vi "DAQ.vi"() -> ()   [LabVIEW 2018]
uses:
  <vilib>/Platform/TimedLoop/XDataNode/timing_clust.ctl
  <vilib>/Platform/TimedLoop/XDataNode/nitl_modes.ctl
  <vilib>/Platform/TimedLoop/XDataNode/wakeup.ctl
  <vilib>/Analysis/baseanly.llb/Mean (DBL).vi
  <vilib>/FPGAPlugInAG/myRIO-1900/niLvFpga_Open_myRIO-1900.vi
  <vilib>/rvi/interface/common/dynamic/niFpgaDynamicAddResources.vi
  <vilib>/Utility/error.llb/Error Cluster From Error Code.vi
  <vilib>/rvi/errors/niLvFpgaAdjustHostInterfaceError.vi
  <vilib>/FPGAPlugInAG/Dynamic/niLvFpga_Close_Dynamic.vi
  <vilib>/rvi/interface/nirviOpenFPGA/nirviOpenFPGA.xnode
  FPGA Bitfiles/FirstTrial_FPGATarget_FPGAMain_Binary_Stochastic_DIO.lvbitx
  <vilib>/rvi/interface/nirviReadWriteControl/nirviReadWriteControl.xnode
  <vilib>/rvi/interface/nirviMethod/nirviMethod.xnode
  <vilib>/Platform/TimedLoop/XDataNode/XDataNode.xnode
  <vilib>/rvi/interface/nirviCloseFPGA/nirviCloseFPGA.xnode
  <vilib>/rvi/errors/niLvFpgaMergeErrorWithErrorCode.vi
  <vilib>/rvi/interface/Simulation/niFpgaSimulationCallBeginRW.vi
  <vilib>/Platform/TimedLoop/XDataNode/XDNodeRunTimeDep.lvlib
  <vilib>/Analysis/NI_AALBase.lvlib
  <vilib>/FPGAPlugInAG/Dynamic/niLvFpga_ReadFifo_Dynamic.vi
  NiFpgaLv.dll
  <vilib>/FPGAPlugInAG/Dynamic/niLvFpga_StartFifo_Dynamic.vi
  <vilib>/FPGAPlugInAG/Dynamic/niLvFpga_StopFifo_Dynamic.vi
panel:
  in  "Acquisitions":T1(tab)=enum."Recorded"
  out "Real Time Actuation Mean Chart":dbl(graph)=2.577495574951172
  out "Real Time Measurement Mean Chart":dbl(graph)=2.4726343154907227
  out "Measurement Data":i16[](array[numeric])=[754, 1268, 1779, 2292, 2798, 3300, 3794, 4083, 4089, 4094, 4094, 4095, 4093, 4095, 4094, 4095, 4094, 4095, 4093, 4095, 4093, 4094, 4093, 4095, 4093, 4095, 4093, 4095, 4093, 4095, 4093, 4095, 4093, 4095, 4093, 4095, 4092, 4095, 4092, 4095, 4092, 4095, 4092, 4095, 4093, 4095, 4094, 4095, 4094, 4095, 4094, 4095, 4094, 4095, 4095, 4095, 4094, 4095, 4094, 4094, 3947, 3428, 2884, 2343, 1812, 1284, 760, 250, 10, 8, 5, 5, 4, 4, 5, 5, 5, 5, 5, 4, 5, 5, 5, 4, 5, 4, 5, 5, 5, 5, 5, 5, 5, 4, 5, 5, 5, 5, 4, 5, 4, 5, 5, 5, 5, 4, 4, 5, 5, 5, 5, 5, 4, 5, 5, 5, 4, 5, 5, 5, 5, 5, 5, 136, 636, 1150, 1662, 2175, 2682, 3186, 3680, 4088, 4089, 4093, 4093, 4095, 4094, 4095, 4093, 4095, 4094, 4095, 4093, 4094, 4093, 4095, 4093, 4094, 4093, 4095, 4093, 4095, 4094, 4095, 4094, 4095, 4093, 4095, 4093, 4095, 4093, 4095, 4092, 4095, 4092, 4095, 4092, 4095, 4093, 4095, 4094, 4095, 4093, 4095, 4094, 4095, 4094, 4095, 4094, 4095, 4094, 4095, 4094, 4095, 4060, 3570, 3029, 2485, 1952, 1423, 897, 382, 4, 9, 6, 5, 4, 4, 5, 5, 5, 5, 4, 4, 4, 5, 5, 4, 5, 5, 5, 5, 5, 5, 5, 5, 4, 5, 5, 5, 5, 5, 5, 4, 5, 5, 5, 4, 4, 4, 5, 5, 5, 5, 5, 5, 5, 5, 5, 5, 5, 4, 5, 5, 5, 5, 5, 7, 500, 1013, 1526, 2037, 2548, 3052, 3550, 4034]
  out "Actuation Data":i16[](array[numeric])=[4095, 4095, 4095, 4095, 4095, 4095, 4095, 4095, 4095, 4095, 4095, 4095, 4095, 4095, 4095, 4095, 4095, 4095, 4095, 4095, 4095, 4095, 4095, 4095, 4095, 4095, 4095, 4095, 4095, 4095, 4095, 4095, 4095, 4095, 4095, 4095, 4095, 4095, 4095, 4095, 4095, 4095, 4095, 4095, 4095, 4095, 4095, 4095, 4095, 4095, 4095, 4095, 4095, 4095, 4095, 4095, 4095, 4095, 4095, 0, 0, 0, 0, 0, 0, 0, 0, 0, 0, 0, 0, 0, 0, 0, 0, 0, 0, 0, 0, 0, 0, 0, 0, 0, 0, 0, 0, 0, 0, 0, 0, 0, 0, 0, 0, 0, 0, 0, 0, 0, 0, 0, 0, 0, 0, 0, 0, 0, 0, 0, 0, 0, 0, 0, 0, 0, 0, 0, 0, 0, 0, 4095, 4095, 4095, 4095, 4095, 4095, 4095, 4095, 4095, 4095, 4095, 4095, 4095, 4095, 4095, 4095, 4095, 4095, 4095, 4095, 4095, 4095, 4095, 4095, 4095, 4095, 4095, 4095, 4095, 4095, 4095, 4095, 4095, 4095, 4095, 4095, 4095, 4095, 4095, 4095, 4095, 4095, 4095, 4095, 4095, 4095, 4095, 4095, 4095, 4095, 4095, 4095, 4095, 4095, 4095, 4095, 4095, 4095, 4095, 4095, 4095, 4095, 0, 0, 0, 0, 0, 0, 0, 0, 0, 0, 0, 0, 0, 0, 0, 0, 0, 0, 0, 0, 0, 0, 0, 0, 0, 0, 0, 0, 0, 0, 0, 0, 0, 0, 0, 0, 0, 0, 0, 0, 0, 0, 0, 0, 0, 0, 0, 0, 0, 0, 0, 0, 0, 0, 0, 0, 0, 0, 0, 0, 0, 0, 4095, 4095, 4095, 4095, 4095, 4095, 4095, 4095, 4095, 4095, 4095]
  out "Mean Measurement":dbl=2.4726343154907227 format="%0.2f"
  out "Mean Acatuation":dbl=2.577495574951172 format="%0.2f"
  out "Elements Remaining":u32=192
  out "Actuation Graph":waveform(i16)(graph)={"t0"=timestamp(0 s since 1904-01-01), "dt"=2.0, "Y"=array[3392 elements]}
  out "Measurement Graph":waveform(i16)(graph)={"t0"=timestamp(0 s since 1904-01-01), "dt"=2.0, "Y"=array[3520 elements]}
  out "Data File Path":path=path "c:/ni-rt/startup/03_11_16_04:11 PMTrial.csv"
  out "Sample Each Cycle":i32[](array[numeric])=[0, 0, 512, 960, 576, 384, 256, 192, 256, 256]
  out "Total Data Points":i32=3392
  in  "Settings":enum32{"Controls", "Logging Setting"}(tab)
  in  "Actuation Period (muS)":u32=5
  in  "Acquisition Period (muS)":u32=2
  in  "RT Period(muS)":i64=500
  in  "Recording Time (muS)":i64=5000
  in  "Signal Control":T2={"Mode"=enum."Square Wave", "Frequency (Periods/tick)"=0.0001005989033728838, "Phase (period)"=0.0} {"Frequency (Periods/tick)" format="%#_6f"}
  out "Frequency (kHz)":dbl=4.023956134915352
  in  "High Pass?":bool
  in  "Low Pass?":bool
  in  "Data File Name Label":string="Trial"
  in  "Continuous?":bool
  in  "Log Data?":bool
  out "Logging Progress":dbl(slide) scale=0.0..100.0
  out "Logging?":bool
  out "Finished Late? [i-1]":bool
  out "FIFO Timed Out?":bool
  in  "stop":bool
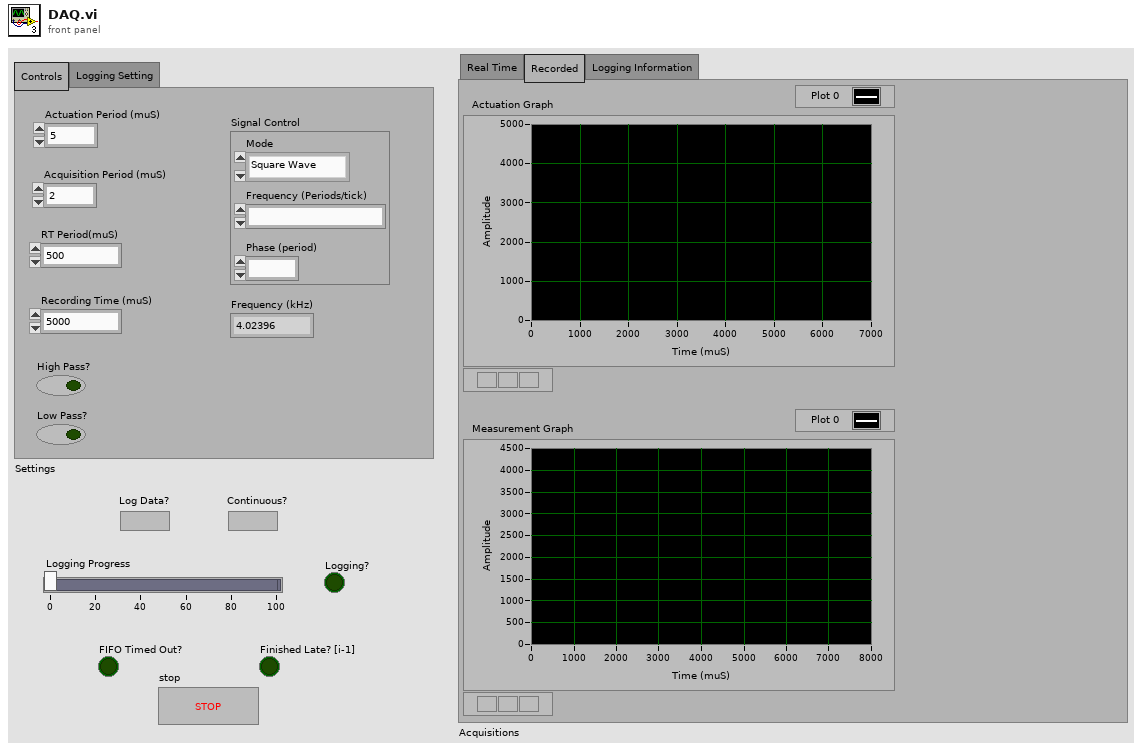
[diagram p1: front panel]
types:
  T1 = enum32{"Real Time", "Recorded", "Logging Information"}
  T2 = cluster{"Mode":enum16{"Square Wave", "Sine Wave", "White Noise", "Stochastic"}, "Frequency (Periods/tick)":fxp<+,32,0>, "Phase (period)":fxp<+,32,0>}
  T3 = typedef "XDNodeRunTimeDep.lvlib/timing_clust.ctl" = cluster{"Expected End [f-1]":u64, "Actual End [f-1]":u64, "Finished Late? [f-1]":bool, "Expected End [i-1]":u64, "Actual End [i-1]":u64, "Finished Late? [i-1]":bool, "Expected Start [i]":u64, "Actual Start [i]":u64, "Expected Start [f]":u64, "Actual Start [f]":u64, "Source Name":string, "Structure Name":string, "Period":i64, "Deadline":i64, "Offset":i64, "Start":i64, "Priority":i32, "Timeout":i32, "Mode":T4, "Wakeup Reason":T5, "Error":errorcluster, "Source Type":string, "Secondary Source Type":string, "Global End Time":u64, "Global Start Time":u64, "Frame Duration":u64, "Iteration Duration":u64, "Assigned CPU":i32, "I/O Scan Engine Mode":u32}
  T4 = typedef "XDNodeRunTimeDep.lvlib/nitl_modes.ctl" = enum32{"No Change", "Process missed periods, maintain original phase", "Discard missed periods, maintain original phase", "Process missed periods, ignore original phase", "Discard missed periods, ignore original phase"}
  T5 = typedef "XDNodeRunTimeDep.lvlib/wakeup.ctl" = enum32{"Normal", "Aborted", "Asynchronous wakeup", "Timing source error", "Timed loop error", "Timeout"}
  T6 = enum16{"open", "replace", "create", "open or create", "replace or create", "replace or create with confirmation"}
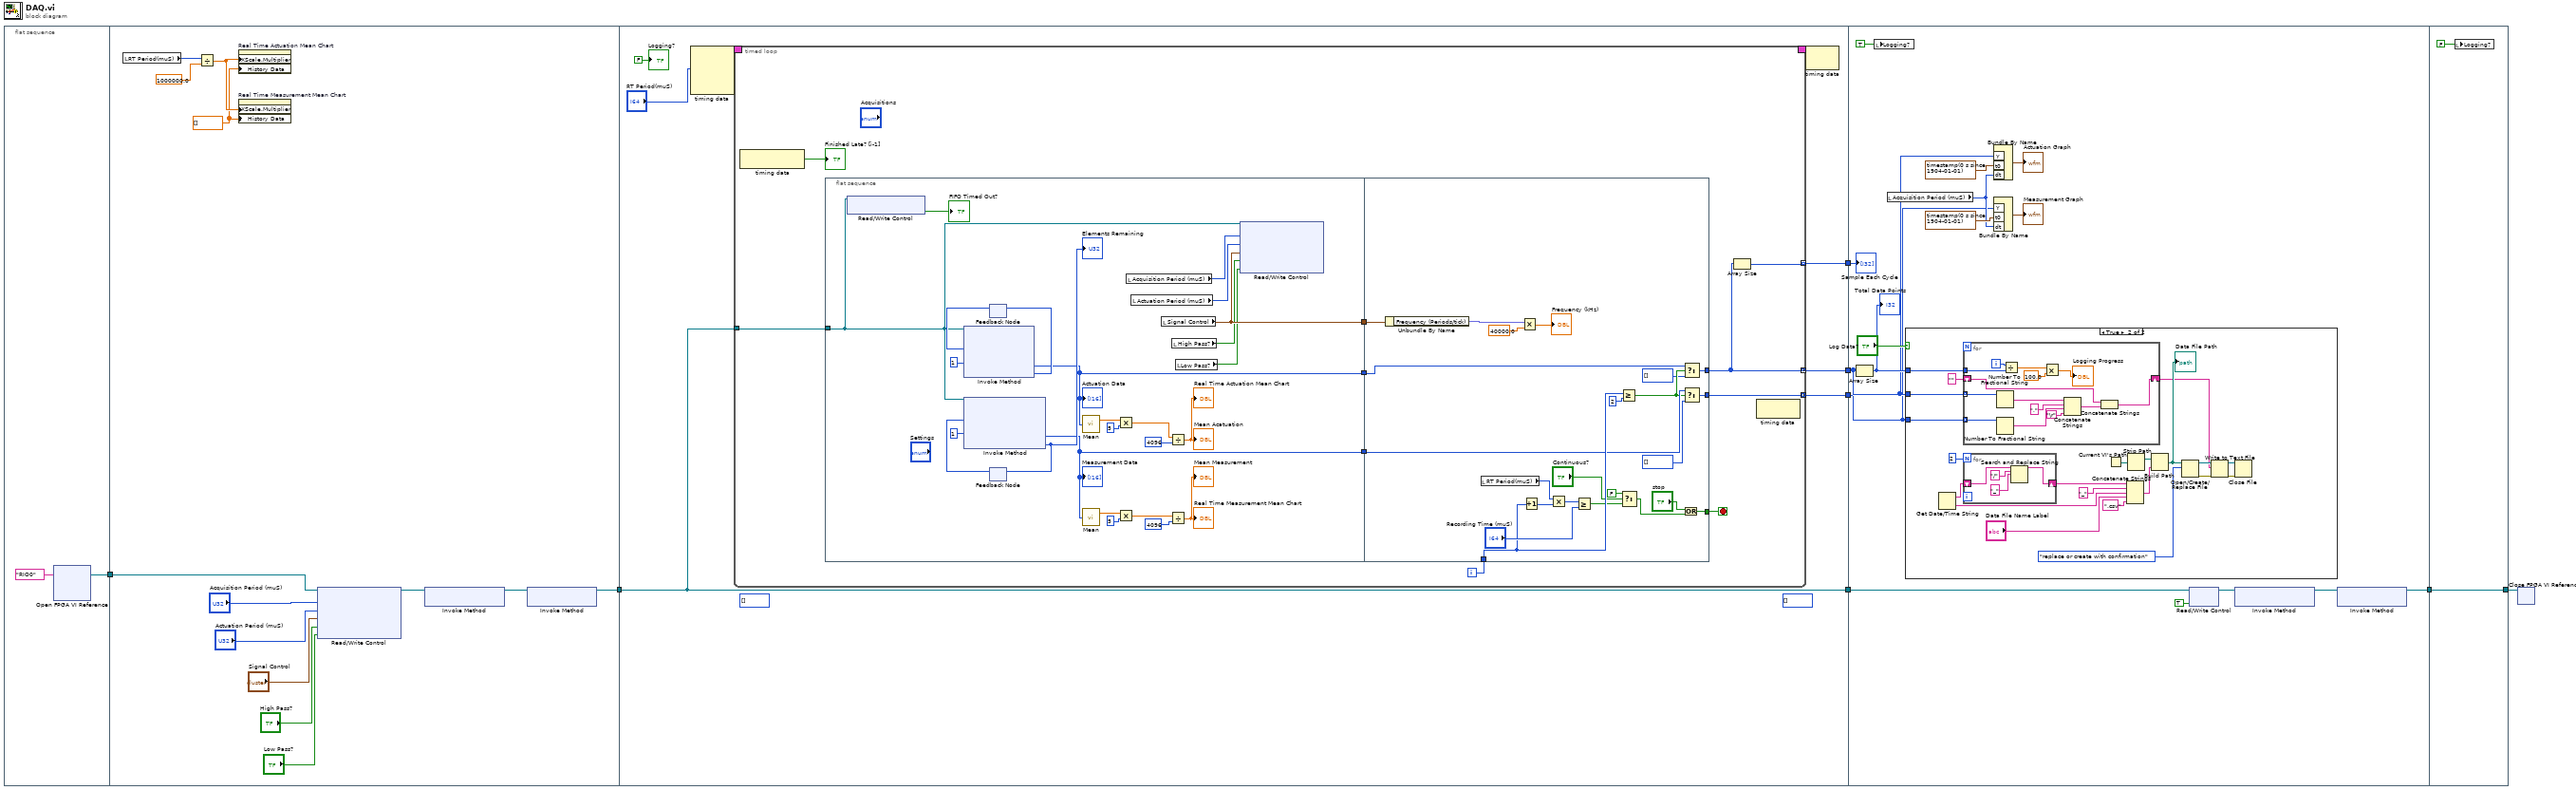
[diagram p0: block diagram]
diagram:
  n1 = flat-sequence {
    tunnel: [w9] -> w6
    tunnel: w6 -> [w16]
    tunnel: [w15] -> w5
    tunnel: w5 -> [w28]
    tunnel: [w28] -> w8
    tunnel: [w27] -> w4
    tunnel: [w26] -> w3
    tunnel: [w24] -> w1
    tunnel: w8 -> [w110]
    tunnel: w4 -> [w102]
    tunnel: w3 -> [w97]
    tunnel: [w111] -> w2
    tunnel: w1 -> [w106]
    tunnel: [w153] -> w7
    tunnel: w2 -> [w153]
    frame #0 {
      n2 = xnode "Open FPGA VI Reference"("resource name"=tag "RIO0") -> ("FPGA VI Reference Out"=w9:refnum<k20>)  [unwired: 1 in, 1 out]
    }
    frame #1 {
      w13 = dbl[] [] ("History Data")
      n3 = local read "RT Period(muS)"() -> (w19:i64)
      n4 = Divide(x=w19, y=1000000.0 ("x")) -> (x/y=w14:dbl)
      n5 = property on="Real Time Actuation Mean Chart" class="WFChart (strict)"("XScale.Multiplier"=w14, "History Data"=w13) -> ()  [unwired: 2 in, 2 out]
      n6 = property on="Real Time Measurement Mean Chart" class="WFChart (strict)"("XScale.Multiplier"=w14, "History Data"=w13) -> ()  [unwired: 2 in, 2 out]
      n7 = xnode "Read/Write Control"("FPGA VI Reference In"=w16, "Acquisition Period (muS)"="Acquisition Period (muS)", "Actuation Period (muS)"="Actuation Period (muS)", "Cluster"="Signal Control", "High Pass?"="High Pass?", "Low Pass?"="Low Pass?") -> ("FPGA VI Reference Out"=w18:refnum<k20>)  [unwired: 1 in, 1 out]
      n8 = xnode "Invoke Method"("FPGA VI Reference In"=w18) -> ("FPGA VI Reference Out"=w17:refnum<k20>)  [unwired: 1 in, 1 out]
      n9 = xnode "Invoke Method"("FPGA VI Reference In"=w17) -> ("FPGA VI Reference Out"=w15:refnum<k20>)  [unwired: 1 in, 1 out]
    }
    frame #2 {
      (unwired) i16[] []
      (unwired) i16[] []
      n10 = node-c288("RT Period(muS)") -> (w31:T3)  [unwired: 3 in]
      n11 = timed-loop {
        tunnel: w28 -> [w40]
        timing: w31 -> [_]
        timing-out: [_] -> w30
        tunnel: [w34] -> w27 mode=concatenating
        tunnel: [w39] -> w26 mode=concatenating
        tunnel: [w33] -> w24 mode=indexing
        i -> [w36]
        stop <- w35 stop-if-true
        n12 = node-c288() -> (→"Finished Late? [i-1]":bool)  [unwired: 1 in]
        n13 = flat-sequence {
          tunnel: w40 -> [w51]
          tunnel: [w48] -> w38
          tunnel: [w47] -> w37
          tunnel: [w44] -> w32
          tunnel: [w83] -> w39
          tunnel: [w76] -> w34
          tunnel: w38 -> [w77]
          tunnel: w37 -> [w80]
          tunnel: w36 -> [w82]
          tunnel: [w84] -> w35
          tunnel: w32 -> [w74]
          frame #0 {
            n14 = xnode "Read/Write Control"("FPGA VI Reference In"=w51) -> ("Acquistion Timed Out?"=→"FIFO Timed Out?":bool)  [unwired: 1 in, 2 out]
            n15 = feedback #1() -> (w57:u32)  [unwired: 1 in]
            n16 = xnode "Invoke Method"("FPGA VI Reference In"=w51, "Number of Elements"=w57, "Timeout (ms)"=1) -> ("Data"=w48:i16[], "Elements Remaining"=w56:u32)  [unwired: 1 in, 2 out]
            "Actuation Data" <- w48
            n17 = feedback-in #1(w56) -> ()
            n18 = feedback #2() -> (w64:u32)  [unwired: 1 in]
            n19 = xnode "Invoke Method"("FPGA VI Reference In"=w51, "Number of Elements"=w64, "Timeout (ms)"=1) -> ("Data"=w47:i16[], "Elements Remaining"=w65:u32)  [unwired: 1 in, 2 out]
            "Measurement Data" <- w47
            "Elements Remaining" <- w65
            n20 = feedback-in #2(w65) -> ()
            n21 = call-poly <vilib>:"Mean.vi"("X"=w48) -> ("mean"=w52:dbl)  [unwired: 1 out]
            n22 = call-poly <vilib>:"Mean.vi"("X"=w47) -> ("mean"=w59:dbl)  [unwired: 1 out]
            n23 = Multiply(x=w52, y=u16 5) -> (x*y=w53:dbl)
            n24 = Multiply(x=w59, y=u16 5) -> (x*y=w60:dbl)
            n25 = local read "Acquisition Period (muS)"() -> (w50:u32)
            n26 = local read "Actuation Period (muS)"() -> (w49:u32)
            n27 = local read "Signal Control"() -> (w44:T2)
            n28 = Divide(x=w53, y=u16 4096) -> (x/y=→"Real Time Actuation Mean Chart" →"Mean Acatuation":dbl)
            n29 = Divide(x=w60, y=u16 4096) -> (x/y=→"Mean Measurement" →"Real Time Measurement Mean Chart":dbl)
            n30 = local read "High Pass?"() -> (w43:bool)
            n31 = local read "Low Pass?"() -> (w42:bool)
            n32 = xnode "Read/Write Control"("FPGA VI Reference In"=w51, "Acquisition Period (muS)"=w50, "Actuation Period (muS)"=w49, "Cluster"=w44, "High Pass?"=w43, "Low Pass?"=w42) -> ()  [unwired: 1 in, 2 out]
          }
          frame #1 {
            n33 = Unbundle By Name(w74) -> ("Frequency (Periods/tick)"=w72:fxp<+,32,0>)
            n34 = local read "RT Period(muS)"() -> (w86:i64)
            n35 = Multiply(x=w72, y=40000.0) -> (x*y=→"Frequency (kHz)":dbl)
            n36 = Increment(x=w82) -> (x+1=w88:i32)
            n37 = Multiply(x=w86, y=w88) -> (x*y=w87:i64)
            n38 = Greater Or Equal?(x=w87, y="Recording Time (muS)") -> (x >= y?=w69:bool)
            n39 = Greater Or Equal?(x=w82, y=2) -> (x >= y?=w78:bool)
            n40 = Select(t=FALSE, s="Continuous?", f=w69) -> (s? t:f=w68:bool)
            n41 = Or(x="stop", y=w68) -> (x .or. y?=w84:bool)
            n42 = Select(t=w77, s=w78, f=i16[] []) -> (s? t:f=w76:i16[])
            n43 = Select(t=w80, s=w78, f=i16[] []) -> (s? t:f=w83:i16[])
          }
        }
        n44 = Array Size(array=w34) -> (size(s)=w33:i32)
        n45 = node-c288() -> ()  [unwired: 1 in, 1 out]
      }
      n46 = node-c288(w30) -> ()  [unwired: 1 out]
      "Logging?" <- FALSE ("Logging?")
    }
    frame #3 {
      n47 = Array Size(array=w102) -> (size(s)=w105:i32)
      "Total Data Points" <- w105
      n48 = local write "Logging?"(TRUE ("Logging?")) -> ()
      n49 = local read "Acquisition Period (muS)"() -> (w98:u32)
      n50 = case shown="True" "Log Data?" {
        tunnel: w97 -> [_ w118]
        tunnel: w102 -> [_ w117]
        tunnel: w105 -> [_ w116]
        frame False {
        }
        frame True {
          n51 = Get Date/Time String() -> (date string=w126:string, time string=w122:string)  [unwired: 3 in]
          n52 = for {
            shift-right: [w144] -> w115
            shift-left: "" -> [w143]
            tunnel: w118 -> [w140] mode=indexing
            tunnel: w117 -> [w139] mode=indexing
            tunnel: w116 -> [w135]
            i -> [w134]
            n53 = Number To Fractional String(number=w139) -> (F-format string=w142:string)  [unwired: 3 in]
            n54 = Number To Fractional String(number=w140) -> (F-format string=w146:string)  [unwired: 3 in]
            n55 = Divide(x=w134, y=w135) -> (x/y=w138:dbl)
            n56 = Multiply(x=w138, y=100.0) -> (x*y=→"Logging Progress":dbl)
            n57 = Concatenate Strings(w142, "," ("string"), w146, "\r") -> (w145:string)
            n58 = Concatenate Strings(w143, w145) -> (w144:string)
          }
          n59 = for {
            N: 2 -> [_]
            shift-right: [w149] -> w124
            shift-left: w126 -> [w148]
            n60 = Search and Replace String(input string=w148, search string="/", replace string="_" ("replace string (\"\")")) -> (result string=w149:string)  [unwired: 5 in, 3 out]
          }
          n61 = Current VI's Path() -> (path=w128:path)
          n62 = Concatenate Strings(w124, "_" ("replace string (\"\")"), w122, "Data File Name Label", ".csv" ("replace string (\"\")")) -> (w121:string)
          n63 = Strip Path(path=w128) -> (stripped path=w127:path)  [unwired: 1 out]
          n64 = Build Path(base path=w127, name or relative path=w121) -> (appended path=w120:path)
          "Data File Path" <- w120
          n65 = Open/Create/Replace File(file path (use dialog)=w120, operation (0:open)=T6."replace or create with confirmation") -> (refnum out=w132:refnum<file>, error out=w131:errorcluster)  [unwired: 4 in, 1 out]
          n66 = Write to Text File(file (use dialog)=w132, text=w115, error in=w131) -> (refnum out=w130:refnum<file>, error out=w129:errorcluster)  [unwired: 1 in, 1 out]
          n67 = Close File(refnum=w130, error in=w129) -> ()  [unwired: 2 out]
        }
      }
      n68 = Bundle By Name("Y"=w102, "t0"=timestamp(0 s since 1904-01-01), "dt"=w98) -> (→"Actuation Graph":waveform(i16))  [unwired: 1 in]
      n69 = Bundle By Name("Y"=w97, "t0"=timestamp(0 s since 1904-01-01), "dt"=w98) -> (→"Measurement Graph":waveform(i16))  [unwired: 1 in]
      n70 = xnode "Read/Write Control"("FPGA VI Reference In"=w110, "stop"=TRUE) -> ("FPGA VI Reference Out"=w109:refnum<k20>)  [unwired: 1 in, 1 out]
      n71 = xnode "Invoke Method"("FPGA VI Reference In"=w109) -> ("FPGA VI Reference Out"=w112:refnum<k20>)  [unwired: 1 in, 1 out]
      n72 = xnode "Invoke Method"("FPGA VI Reference In"=w112) -> ("FPGA VI Reference Out"=w111:refnum<k20>)  [unwired: 1 in, 1 out]
      "Sample Each Cycle" <- w106
    }
    frame #4 {
      n73 = local write "Logging?"(FALSE ("Logging?")) -> ()
    }
  }
  n74 = xnode "Close FPGA VI Reference"("FPGA VI Reference In"=w7) -> ()  [unwired: 1 in, 1 out]
